vi "Top.vi"(8 "error in (no error)":errorcluster, 9 "reposition window":bool, 10 "window position":cluster{"Left":i16, "Top":i16}, 11 "Thread in":refnum<class "Thread.lvclass">) -> (0 "error":errorcluster, 3 "Thread out":refnum<class "Thread.lvclass">)   [LabVIEW 2019, in "DSF Core.lvlib" / "Thread.lvclass"]
uses:
  Thread.lvclass
  <vilib>/Platform/TimedLoop/XDataNode/wakeup.ctl
  <vilib>/Platform/TimedLoop/XDataNode/XDNodeRunTimeDep.lvlib
  <vilib>/Platform/TimedLoop/XDataNode/nitl_modes.ctl
  <vilib>/Platform/TimedLoop/XDataNode/timing_clust.ctl
  <vilib>/platform/TimedLoop/XDataNode/XDataNode.xnode
  Thread State.ctl
panel:
  out "Error Count":i32
  out "Priority":u16
  out "Processor":i32
  out "Run Count":i32
  out "State":T1
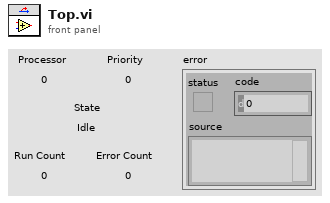
[diagram p1: front panel]
types:
  T1 = typedef "DSF Core.lvlib/Thread.lvclass/Thread State.ctl" = enum8{"Idle", "Running", "Error", "Shut Down"}
  T2 = typedef "XDNodeRunTimeDep.lvlib/timing_clust.ctl" = cluster{"Expected End [f-1]":u64, "Actual End [f-1]":u64, "Finished Late? [f-1]":bool, "Expected End [i-1]":u64, "Actual End [i-1]":u64, "Finished Late? [i-1]":bool, "Expected Start [i]":u64, "Actual Start [i]":u64, "Expected Start [f]":u64, "Actual Start [f]":u64, "Source Name":string, "Structure Name":string, "Period":i64, "Deadline":i64, "Offset":i64, "Start":i64, "Priority":i32, "Timeout":i32, "Mode":T3, "Wakeup Reason":T4, "Error":errorcluster, "Source Type":string, "Secondary Source Type":string, "Global End Time":u64, "Global Start Time":u64, "Frame Duration":u64, "Iteration Duration":u64, "Assigned CPU":i32, "I/O Scan Engine Mode":u32}
  T3 = typedef "XDNodeRunTimeDep.lvlib/nitl_modes.ctl" = enum32{"No Change", "Process missed periods, maintain original phase", "Discard missed periods, maintain original phase", "Process missed periods, ignore original phase", "Discard missed periods, ignore original phase"}
  T4 = typedef "XDNodeRunTimeDep.lvlib/wakeup.ctl" = enum32{"Normal", "Aborted", "Asynchronous wakeup", "Timing source error", "Timed loop error", "Timeout"}
  T5 = typedef "DSF Core.lvlib/Thread.lvclass/Thread Command.ctl" = enum8{"Run", "Shutdown"}
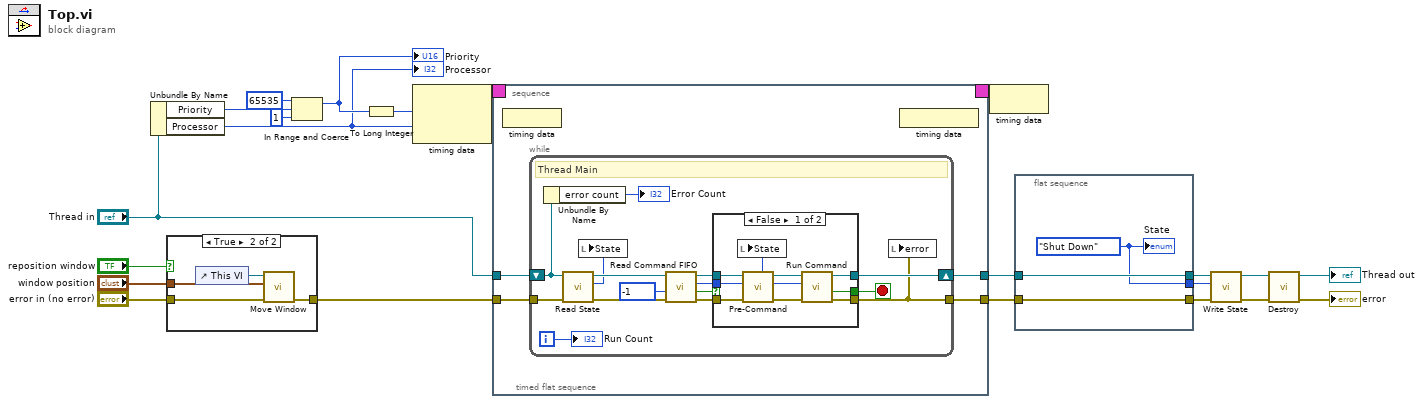
[diagram p0: block diagram]
diagram:
  n1 = Unbundle By Name("Thread in") -> ("Priority"=w12:u16, "Processor"=w5:i32)
  "Processor" <- w5
  n2 = case shown="True" "reposition window" {
    tunnel: "window position" -> [_ w27]
    tunnel: [w23 w25] -> w1
    tunnel: "error in (no error)" -> [w23 w24]
    frame False {
    }
    frame True {
      n3 = control-ref of="This VI"() -> (w26:refnum<vi>)
      n4 = call "Move Window.vi"("error in (no error)"=w24, "window position"=w27, "VI Ref"=w26) -> ("error out"=w25:errorcluster)  [unwired: 8 in]
    }
  }
  n5 = In Range and Coerce(upper limit=u16 65535, x=w12, lower limit=u16 1) -> (coerced(x)=w6:u16)  [unwired: 1 out]
  "Priority" <- w6
  n6 = To Long Integer(number=w6) -> (32bit integer=w15:i32)
  n7 = node-c288(w15, w5) -> (w22:T2)
  n8 = timed-sequence {
    timing: w22 -> [_]
    timing-out: [_] -> w21
    tunnel: [w31] -> w18
    tunnel: [w30] -> w19
    tunnel: "Thread in" -> [w29]
    tunnel: w1 -> [w28]
    n9 = timed-flat-sequence {
      tunnel: [w35] -> w31
      tunnel: [w34] -> w30
      tunnel: w29 -> [w33]
      tunnel: w28 -> [w32]
      n10 = node-c288() -> ()  [unwired: 1 in]
      n11 = while {
        shift-right: [w45] -> w34
        shift-left: w33 -> [w39]
        tunnel: w32 -> [w43]
        tunnel: [w44] -> w35
        i -> [w47]
        stop <- w48 stop-if-true
        # "Thread Main"
        n12 = Unbundle By Name(w39) -> ("error count"=→"Error Count":i32)
        n13 = call "Read State.vi"("error in (no error)"=w43, "Thread in"=w39) -> ("error out"=w41:errorcluster, "state"=w40:T1, "Thread out"=w42:refnum<class "Thread.lvclass">)  [unwired: 7 in]
        n14 = local write "State"(w40) -> ()
        n15 = call "Read Command FIFO.vi"("error in (no error)"=w41, "timeout in ms (0)"=-1, "Thread in"=w42) -> ("error out"=w51:errorcluster, "timed out?"=w49:bool, "command"=w50:T5, "Thread out"=w52:refnum<class "Thread.lvclass">)  [unwired: 4 in, 1 out]
        n16 = case shown="False" w49 {
          selector: w49 -> [_ w63]
          tunnel: [w62 w64] -> w44
          tunnel: [w61 w65] -> w45
          tunnel: w52 -> [w58 w65]
          tunnel: w51 -> [w59 w64]
          tunnel: w50 -> [w57 _]
          tunnel: [w60 w63] -> w48
          frame False {
            n17 = call "Pre-Command.vi"("error in (no error)"=w59, "command in"=w57, "Thread in"=w58) -> ("error out"=w54:errorcluster, "command out"=w56:T5, "Thread out"=w55:refnum<class "Thread.lvclass">, "state"=w53:T1)  [unwired: 5 in]
            n18 = local write "State"(w53) -> ()
            n19 = call "Run Command.vi"("error in (no error)"=w54, "command"=w56, "Thread in"=w55) -> ("error out"=w62:errorcluster, "shutdown?"=w60:bool, "Thread out"=w61:refnum<class "Thread.lvclass">)  [unwired: 6 in]
          }
          frame True {
          }
        }
        n20 = local write "error"(w44) -> ()
        "Run Count" <- w47
      }
      n21 = node-c288() -> ()  [unwired: 1 out]
    }
  }
  n22 = node-c288(w21) -> ()
  n23 = flat-sequence {
    tunnel: [w66] -> w20
    tunnel: w19 -> [w67]
    tunnel: w18 -> [w68]
    tunnel: [w68] -> w17
    tunnel: [w67] -> w16
    frame #0 {
      w66 = Thread_State."Shut Down" ("state")
      "State" <- w66
    }
  }
  n24 = call "Write State.vi"("error in (no error)"=w17, "state"=w20, "Thread in"=w16) -> ("error out"=w10:errorcluster, "Thread out"=w11:refnum<class "Thread.lvclass">)  [unwired: 7 in]
  n25 = call-dynamic "Destroy.vi"("error in (no error)"=w10, "Thread"=w11) -> ("error out"=→"error":errorcluster, "Thread type"=→"Thread out":refnum<class "Thread.lvclass">)  [unwired: 8 in]
